vi "FTW-CodeGen-JSON-GenerateCode.vi"(0 "State In":T2, 5 "XRef":refnum<vi>, 7 "Diagram":refnum<vi>, 9 "Terms":T1(array[cluster])) -> (4 "State Out":T2, 6 "Reply":string[](array[string]), 8 "Generated Code?":bool)   [LabVIEW 2012, in "FTW-JSON-Deserialize.xnode"]
uses:
  src/JSON/FTW-JSON-Deserialize.xnode
  FTW-CodeGen-JSON-State.ctl
  <vilib>/Utility/miscctls.llb/LVPositionTypeDef.ctl
panel:
  # "Inputs"
  # "Outputs"
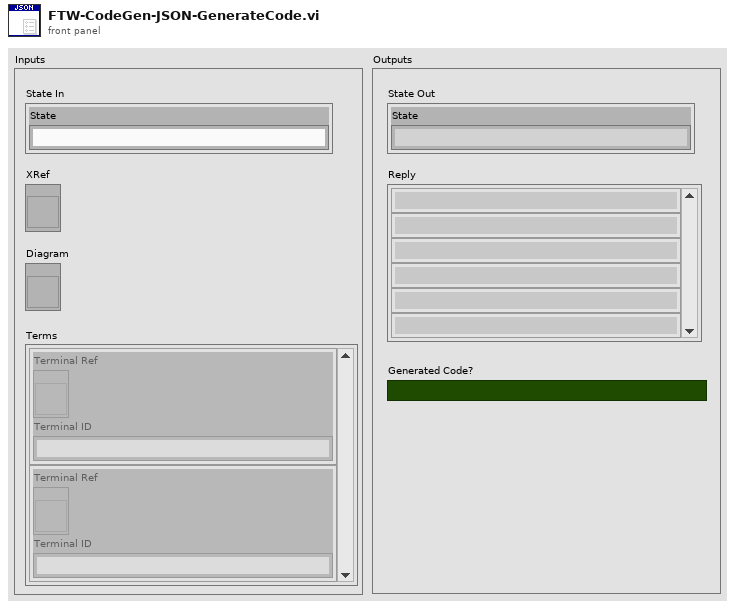
[diagram p1: front panel]
types:
  T1 = cluster{"Terminal Ref":refnum<vi>, "Terminal ID":string}[]
  T2 = typedef "FTW-JSON-Deserialize.xnode/FTW-CodeGen-JSON-State.ctl" = cluster{"State":string}
  T3 = typedef "LVPositionTypeDef.ctl" = cluster{"Left":i32, "Top":i32}
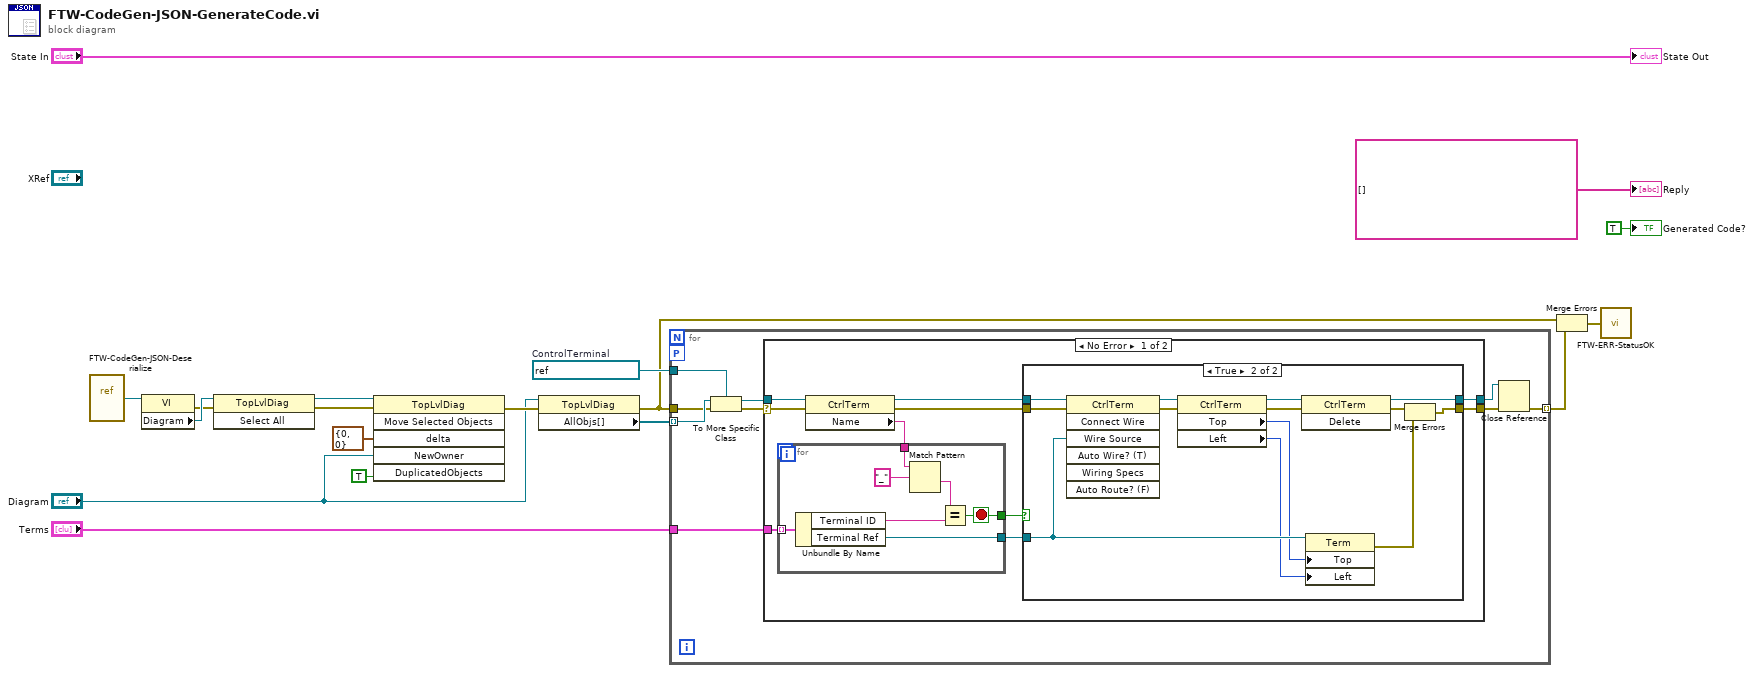
[diagram p0: block diagram]
diagram:
  w11 = refnum<vi> refnum  # ControlTerminal
  n1 = vi-ref "FTW-CodeGen-JSON-Deserialize.vi"() -> (w18:refnum<vi>)
  n2 = property class="VI"(reference=w18) -> (error out=w3:errorcluster, "Diagram"=w9:refnum<vi>)  [unwired: 1 in, 1 out]
  n3 = invoke class="TopLvlDiag" method="Select All"(reference=w9, error in=w3) -> (reference out=w15:refnum<vi>, error out=w14:errorcluster)  [unwired: 1 in, 1 out]
  n4 = invoke class="TopLvlDiag" method="Move Selected Objects"(reference=w15, error in=w14, "delta"=T3 {"Left"=0, "Top"=0} ("position"), "NewOwner"="Diagram", "DuplicatedObjects"=TRUE ("Duplicate? (F)")) -> (error out=w13:errorcluster)  [unwired: 1 in, 5 out]
  n5 = property class="TopLvlDiag"(reference="Diagram", error in=w13) -> (error out=w7:errorcluster, "AllObjs[]"=w12:refnum<vi>[])  [unwired: 1 out]
  n6 = for {
    tunnel: w12 -> [w27] mode=indexing
    tunnel: w7 -> [w26]
    tunnel: w11 -> [w25]
    tunnel: "Terms" -> [w22]
    tunnel: [w19] -> w8 mode=indexing
    workers-P: _ -> [_]
    n7 = To More Specific Class(target class=w25, reference=w27, error in=w26) -> (specific class reference=w23:refnum<vi>, error out=w24:errorcluster)
    n8 = case shown="No Error" w24 {
      selector: w24 -> [w36 _]
      tunnel: w23 -> [w37 w60]
      tunnel: w22 -> [w35 _]
      tunnel: [w28 w60] -> w21
      tunnel: [w29 _] -> w20
      frame No Error {
        n9 = property class="CtrlTerm"(reference=w37, error in=w36) -> (reference out=w32:refnum<vi>, error out=w31:errorcluster, "Name"=w34:string)
        n10 = for {
          tunnel: w35 -> [w59] mode=indexing
          tunnel: w34 -> [w57]
          tunnel: [w58] -> w33
          tunnel: [w53] -> w30
          stop <- w53 stop-if-true
          n11 = Unbundle By Name(w59) -> ("Terminal ID"=w54:string, "Terminal Ref"=w58:refnum<vi>)
          n12 = Match Pattern(string=w57, regular expression="_") -> (after substring=w55:string)  [unwired: 1 in, 3 out]
          n13 = Equal?(x=w55, y=w54) -> (x = y?=w53:bool)
        }
        n14 = case shown="True" w30 {
          tunnel: w33 -> [_ w49]
          tunnel: w32 -> [w39 w52]
          tunnel: [w39 w50] -> w28
          tunnel: w31 -> [w38 w51]
          tunnel: [w38 w41] -> w29
          frame False {
          }
          frame True {
            n15 = invoke class="CtrlTerm" method="Connect Wire"(reference=w52, error in=w51, "Wire Source"=w49) -> (reference out=w48:refnum<vi>, error out=w46:errorcluster)  [unwired: 4 in, 5 out]
            n16 = property class="CtrlTerm"(reference=w48, error in=w46) -> (reference out=w47:refnum<vi>, error out=w45:errorcluster, "Top"=w44:i32, "Left"=w43:i32)
            n17 = invoke class="CtrlTerm" method="Delete"(reference=w47, error in=w45) -> (reference out=w50:refnum<vi>, error out=w42:errorcluster)  [unwired: 1 in, 1 out]
            n18 = property class="Term"(reference=w49, "Top"=w44, "Left"=w43) -> (error out=w40:errorcluster)  [unwired: 1 in, 1 out]
            n19 = Merge Errors(w42, w40) -> (w41:errorcluster)
          }
        }
      }
      frame Error {
      }
    }
    n20 = Close Reference(reference=w21, error in (no error)=w20) -> (error out=w19:errorcluster)
  }
  n21 = Merge Errors(w7, w8) -> (w6:errorcluster)
  n22 = call "FTW-ERR-StatusOK.vi"("error to check"=w6) -> ()  [unwired: 1 out]
  "State Out" <- "State In"
  "Reply" <- string[] [] ("Reply")
  "Generated Code?" <- TRUE ("Generated Code?")
